vi "扫频输出.vi"() -> ()   [LabVIEW 2010]
doc: "I. Description:\nThis example demonstrates how to continuously output a waveform using an internal sample clock. The update rate can be changed while the continuous generation is taking place.\n\nII. Instructions for Running:\n1. Select the Physical Channel to correspond to where your signal is output on the DAQ device.\n2. Enter the Minimum and Maximum Voltage ranges.\n3. Specify the Desired Frequency of the output Waveform. This control can be modified while the generation is taking place.\n4. Enter the Waveform Information. See the documentation of the Waveform Buffer Generation SubVI for information on each parameter.\n\nIII. Block Diagram Steps:\n1. Create an Analog Output Voltage Channel\n2. Call the DAQmx (Sample Clock) VI which sets the sample clock rate based on the rate calculated in the Waveform Buffer Generation subVI. Additionally, set the sample mode to Continuous.\n3. Write the waveform to the output buffer.\n4. Call the Start VI.\n5. Obtain the current value of the Desired Frequency control using a local variable.\n6. Set the sample clock rate to the current desired frequency value using the Waveform Buffer Generation subVI. The Loop runs continuously until user presses the Stop button or an error occurs. Check for errors every 100 ms using the Is Task Done? VI\n7. Call the Clear Task VI to clear the Task.\n8. Use the popup dialog box to display an error or warning if any.\n\nIV. I/O Connections Overview:\nMake sure your signal output terminal matches the Physical Channel I/O Control. For further connection information, refer to your hardware reference manual."
uses:
  <vilib>/Utility/error.llb/DialogType.ctl
  <vilib>/DAQmx/write.llb/DAQmx Write (Analog 1D Wfm NChan NSamp).vi
  <vilib>/DAQmx/create/channels.llb/DAQmx Create Channel (AO-Voltage-Basic).vi
  <vilib>/DAQmx/configure/timing.llb/DAQmx Timing (Sample Clock).vi
  <vilib>/daqmx/miscellaneous.llb/DAQmx Fill In Error Info.vi
  频率.vi
  C:/Program Files/National Instruments/LabVIEW 2010/resource/objmgr/daqmx.rc
panel:
  in  "快扫频间隔(ms)":i32(slide)=250 min=250 max=10000 step=10 scale=0.0..1000.0
  in  "扫频方式\n手动  自动":bool
  in  "一    阶":dbl=14.0
  in  "y 2":dbl=28.0
  in  "二    阶":dbl=131.0
  in  "y 4":dbl=145.0
  in  "慢扫频间隔(ms)":i32(slide)=5000 min=250 max=10000 step=10 scale=0.0..5000.0
  in  "Desired Frequency":dbl=82.0 caption="频率设置" format="%.2f"
  in  "stop":bool
  # "扫频仪"
  # "慢扫频\n\n区    间"
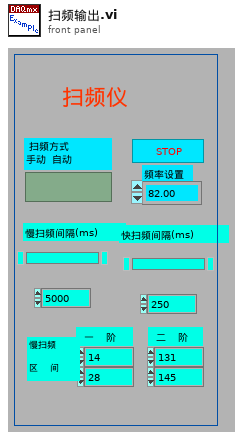
[diagram p1: front panel]
types:
  T1 = enum16{"Sine Wave", "Triangle Wave", "Square Wave", "Sawtooth Wave"}
  T2 = typedef "DialogType.ctl" = u16
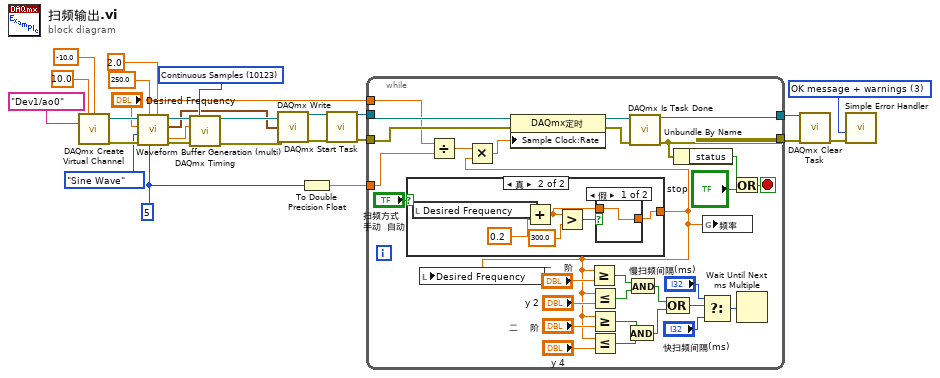
[diagram p0: block diagram]
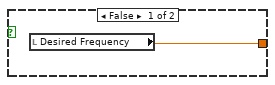
[diagram p2: hidden frame]
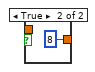
[diagram p3: hidden frame]
diagram:
  w3 = 5 ("Cycles per Buffer")
  w5 = 250.0 ("Samples per Buffer")
  w17 = T2 3 items=["no dialog", "OK message", "continue or stop message", "OK message + warnings", "continue/stop + warnings"] ("type of dialog (OK msg:1)")
  w25 = 10123 items=["Finite Samples"=10178, "Continuous Samples"=10123] ("sample mode")
  n1 = call-poly <vilib>:"DAQmx Create Virtual Channel.vi"("maximum value"=10.0 ("Maximum Value"), "minimum value"=-10.0 ("Minimum Value"), "physical channels"=tag "Dev1/ao0" ("Physical Channels")) -> ("task out"=w12:refnum<k21>, "error out"=w9:errorcluster)  [unwired: 11 in]
  n2 = call "Waveform Buffer Generation (multi).vi"("Amplitude"=2.0, "Cycles per Buffer"=w3, "Samples per Buffer"=w5, "error in (no error)"=w9, "Waveform Type"=T1."Sine Wave", "Desired Frequency"="Desired Frequency", "task/channels in"=w12) -> ("error out"=w10:errorcluster, "Waveform"=w2:waveform(dbl)[], "task out"=w11:refnum<k21>, "Resulting Sample Clock Rate"=w6:dbl)  [unwired: 1 out]
  n3 = call-poly <vilib>:"DAQmx Timing.vi"("task/channels in"=w11, "sample mode"=w25, "rate"=w6, "error in"=w10) -> ("task out"=w18:refnum<k21>, "error out"=w13:errorcluster)  [unwired: 10 in]
  n4 = call-poly <vilib>:"DAQmx Write.vi"("task/channels in"=w18, "data"=w2, "error in"=w13) -> ("task out"=w22:refnum<k21>, "error out"=w21:errorcluster)  [unwired: 10 in, 1 out]
  n5 = To Double Precision Float(number=w3) -> (double precision float=w1:dbl)
  n6 = call <vilib>:"DAQmx Start Task.vi"("task/channels in"=w22, "error in"=w21) -> ("task out"=w26:refnum<k21>, "error out"=w20:errorcluster)  [unwired: 12 in]
  n7 = while {
    tunnel: w26 -> [w47]
    tunnel: [w51] -> w15
    tunnel: w20 -> [w46]
    tunnel: [w52] -> w14
    tunnel: w5 -> [w45]
    tunnel: w1 -> [w50]
    stop <- w55 stop-if-true
    n8 = case shown="真" "扫频方式\n手动  自动" {
      tunnel: [w56 w58] -> w27
      frame False {
        n9 = local read "Desired Frequency"() -> (w56:dbl)
      }
      frame True {
        n10 = local read "Desired Frequency"() -> (w62:dbl)
        n11 = Add(x=w62, y=0.2) -> (x+y=w57:dbl)
        n12 = Greater?(x=w57, y=300.0) -> (0:w60:bool)
        n13 = case shown="假" w60 {
          tunnel: [w63 8] -> w58
          tunnel: w57 -> [w63 _]
          frame False {
          }
          frame True {
          }
        }
      }
    }
    n14 = local write "Desired Frequency"(w27) -> ()
    n15 = Divide(x=w45, y=w50) -> (x/y=w28:dbl)
    n16 = Multiply(x=w28, y=w27) -> (x*y=w44:dbl)
    n17 = property class="DAQmx定时"(reference=w47, error in=w46, "Sample Clock:Rate"=w44) -> (reference out=w49:refnum<k21>, error out=w48:errorcluster)
    n18 = Greater Or Equal?(x=w27, y="一    阶") -> (x >= y?=w38:bool)
    n19 = Less Or Equal?(x=w27, y="y 2") -> (x <= y?=w39:bool)
    n20 = Greater Or Equal?(x=w27, y="二    阶") -> (x >= y?=w40:bool)
    n21 = Less Or Equal?(x=w27, y="y 4") -> (x <= y?=w41:bool)
    n22 = And(x=w40, y=w41) -> (x .and. y?=w43:bool)
    n23 = And(x=w38, y=w39) -> (x .and. y?=w42:bool)
    n24 = call <vilib>:"DAQmx Is Task Done.vi"("task/channels in"=w49, "error in"=w48) -> ("task out"=w51:refnum<k21>, "error out"=w52:errorcluster)  [unwired: 11 in, 1 out]
    n25 = Compound Arithmetic op=OR(w42, w43) -> (w33:bool)
    n26 = Unbundle By Name(w52) -> ("status"=w53:bool)
    n27 = Select(t="慢扫频间隔(ms)", s=w33, f="快扫频间隔(ms)") -> (s? t:f=w30:i32)
    n28 = global write "频率.vi" "频率"(w27) -> ()
    n29 = Or(x=w53, y="stop") -> (x .or. y?=w55:bool)
    n30 = Wait Until Next ms Multiple(millisecond multiple=w30) -> ()  [unwired: 1 out]
  }
  n31 = call <vilib>:"DAQmx Clear Task.vi"("task in"=w15, "error in"=w14) -> ("error out"=w16:errorcluster)  [unwired: 13 in]
  n32 = call <vilib>:"Simple Error Handler.vi"("type of dialog (OK msg:1)"=w17, "error in (no error)"=w16) -> ()  [unwired: 3 in, 5 out]
